vi "RecordAudioSend.vi"(8 "error in (no error)":errorcluster, 10 "audio record cfg":T1, 11 "Qbus in":refnum<class "Qbus.lvclass">) -> (0 "error out":errorcluster, 3 "Qbus out":refnum<class "Qbus.lvclass">)   [LabVIEW 2017, in "EmsaAcquisition.lvlib"]
uses:
  <vilib>/addons/InsightCM/Devices/Shared/Emsa/EmsaAcquisition/EmsaAcquisition.lvlib
  <vilib>/addons/Qbus/Qbus.lvclass
  <vilib>/addons/InsightCM/Devices/Shared/Emsa/EmsaAcquisition/controls/StartOnDemandAcquisitionRoutedMessage.ctl
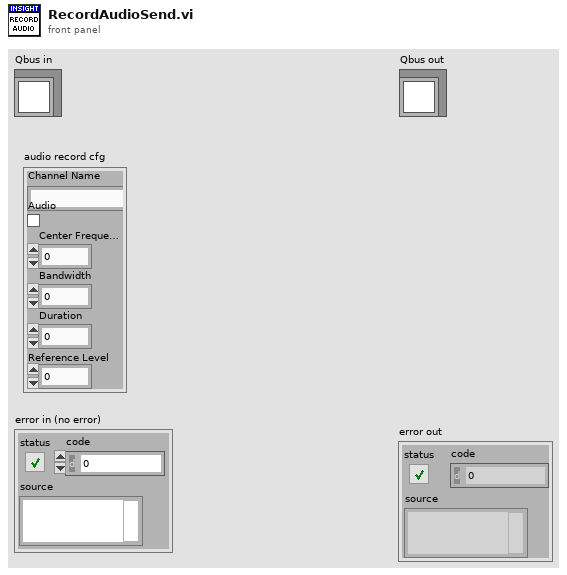
[diagram p1: front panel]
types:
  T1 = typedef "EmsaAcquisition.lvlib/StartOnDemandAcquisitionRoutedMessage.ctl" = cluster{"Channel Name":string, "Audio":bool, "Center Frequency":dbl, "Bandwidth":dbl, "Duration":dbl, "Reference Level":dbl}
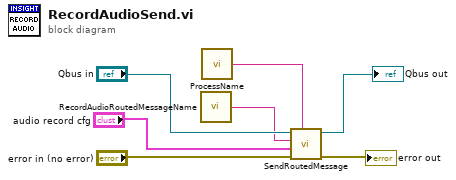
[diagram p0: block diagram]
diagram:
  n1 = call <vilib>:"RecordAudioRoutedMessageName.vi"() -> ("message name"=w2:string)  [unwired: 5 in]
  n2 = call <vilib>:"ProcessName.vi"() -> ("process name"=w1:string)  [unwired: 5 in]
  n3 = call <vilib>:"SendRoutedMessage.vi"("listener process"=w1, "error in (no error)"="error in (no error)", "message value"="audio record cfg", "message name"=w2, "Qbus in"="Qbus in") -> ("error in (no error)"=→"error out":errorcluster, "Qbus out"=→"Qbus out":refnum<class "Qbus.lvclass">)  [unwired: 5 in]
